vi "DriveStraightPECommand.vi"(9 "Fwd Bwd":dbl, 10 "Delay ms":u32=500, 11 "distance":dbl) -> ()   [LabVIEW 2014]
uses:
  Robot Global Data.vi
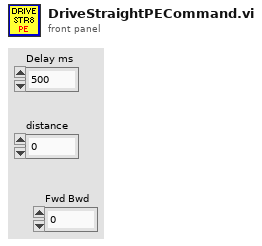
[diagram p1: front panel]
types:
  T1 = typedef "WPI_EncoderDevRef.ctl" = cluster{"DevStatus":errorcluster, "EncoderIndex":T2, "CounterIndex":T3, "DistancePerCount":dbl, "Decoding Type":T4}
  T2 = typedef "FPGA_EncoderIdx.ctl" = enum8{"Enc 0", "Enc 1", "Enc 2", "Enc 3", "Enc 4", "Enc 5", "Enc 6", "Enc 7", "Invalid"}
  T3 = typedef "FPGA_CounterCtrSystemIndex.ctl" = enum8{"Ctr 0", "Ctr 1", "Ctr 2", "Ctr 3", "Ctr 4", "Ctr 5", "Ctr 6", "Ctr 7", "Invalid"}
  T4 = typedef "WPI_EncoderType.ctl" = enum16{"1x", "2x", "4x"}
  T5 = typedef "WPI_GyroDevRef.ctl" = cluster{"DevStatus":errorcluster, "Analog Module":T6, "Analog Channel":T7, "Offset":dbl, "Gain (VoltsPerDegree/Second)":dbl}
  T6 = typedef "FPGA_TypedefAnalogModule.ctl" = enum16{"Controller 1"}
  T7 = typedef "FPGA_AIChannel.ctl" = enum8{"AI 0", "AI 1", "AI 2", "AI 3", "AI MXP 0", "AI MXP 1", "AI MXP 2", "AI MXP 3", "Invalid"}
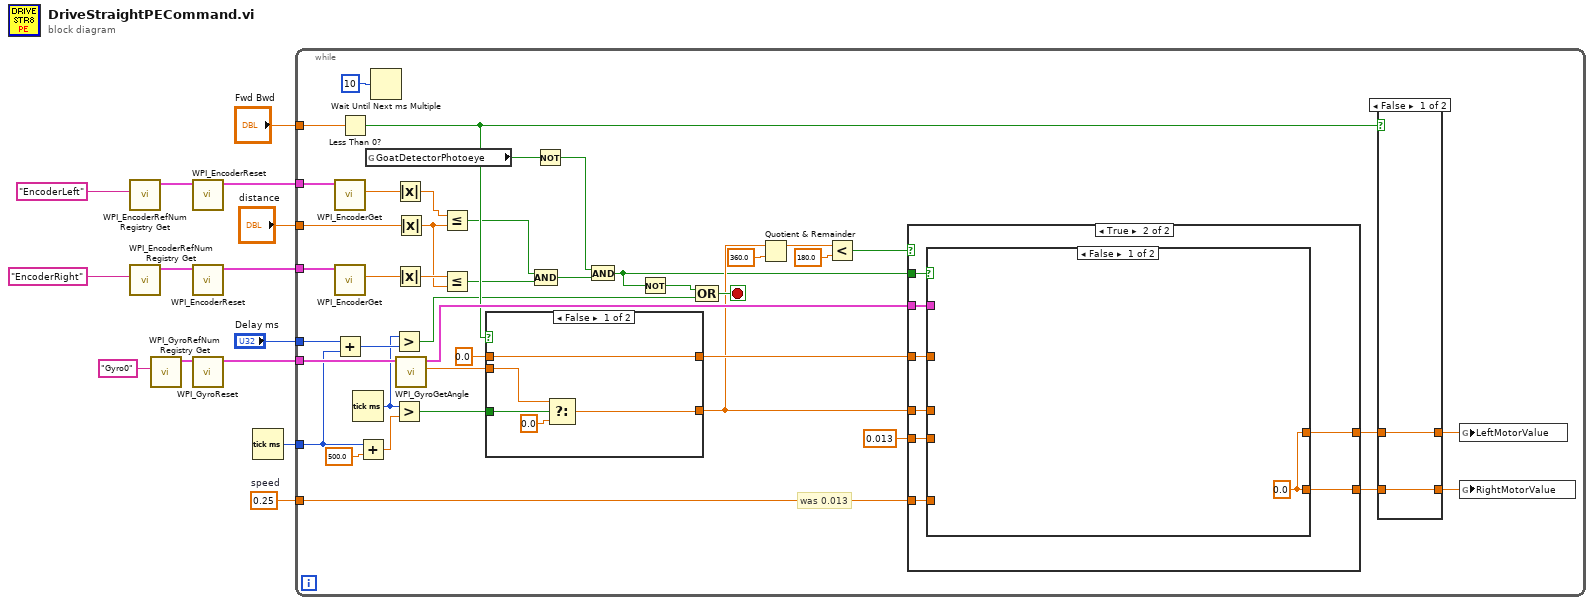
[diagram p0: block diagram]
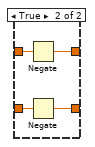
[diagram p2: hidden frame]
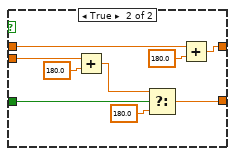
[diagram p3: hidden frame]
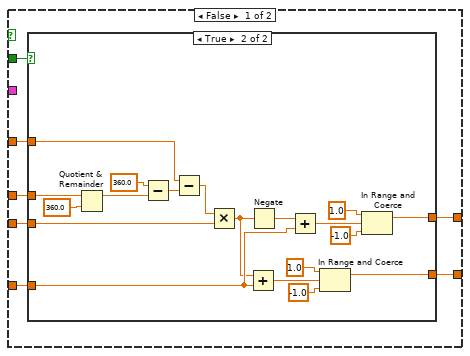
[diagram p4: hidden frame]
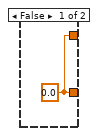
[diagram p5: hidden frame]
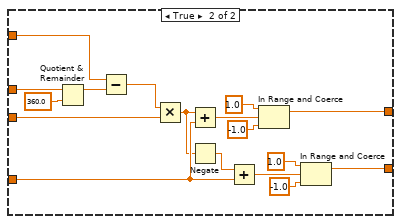
[diagram p6: hidden frame]
diagram:
  w3 = 0.25  # speed
  n1 = call <vilib>:"WPI_EncoderRefNum Registry Get.vi"("refnum name"="EncoderLeft") -> ("EncoderDevRef"=w13:T1)  [unwired: 9 in, 1 out]
  n2 = call <vilib>:"WPI_EncoderRefNum Registry Get.vi"("refnum name"="EncoderRight") -> ("EncoderDevRef"=w12:T1)  [unwired: 9 in, 1 out]
  n3 = call <vilib>:"WPI_GyroRefNum Registry Get.vi"("refnum name"="Gyro0") -> ("GyroDevRef"=w5:T5)  [unwired: 9 in, 1 out]
  n4 = call <vilib>:"WPI_EncoderReset.vi"("EncoderDevRef"=w13) -> ("EncoderDevRef"=w8:T1)  [unwired: 9 in, 1 out]
  n5 = call <vilib>:"WPI_EncoderReset.vi"("EncoderDevRef"=w12) -> ("EncoderDevRef"=w7:T1)  [unwired: 9 in, 1 out]
  n6 = call <vilib>:"WPI_GyroReset.vi"("GyroDevRef"=w5) -> ("GyroDevRef"=w4:T5)  [unwired: 9 in, 1 out]
  n7 = Tick Count (ms)() -> (millisecond timer value=w1:u32)
  n8 = while {
    tunnel: w3 -> [w50]
    tunnel: "distance" -> [w38]
    tunnel: w4 -> [w44]
    tunnel: w8 -> [w43]
    tunnel: w7 -> [w42]
    tunnel: "Fwd Bwd" -> [w41]
    tunnel: "Delay ms" -> [w27]
    tunnel: w1 -> [w25]
    stop <- w39 stop-if-true
    # "was 0.013"
    n9 = call <vilib>:"WPI_EncoderGet.vi"("EncoderDevRef"=w43) -> ("Distance"=w51:dbl)  [unwired: 5 in, 5 out]
    n10 = call <vilib>:"WPI_EncoderGet.vi"("EncoderDevRef"=w42) -> ("Distance"=w55:dbl)  [unwired: 5 in, 5 out]
    n11 = Add(x=w27, y=w25) -> (x+y=w29:u32)
    n12 = Less Than 0?(x=w41) -> (x < 0?=w35:bool)
    n13 = Tick Count (ms)() -> (millisecond timer value=w23:u32)
    n14 = Add(x=w25, y=500.0) -> (x+y=w24:dbl)
    n15 = global read "Robot Global Data.vi" "GoatDetectorPhotoeye"() -> (w21:bool)
    n16 = Wait Until Next ms Multiple(millisecond multiple=u32 10 ("milliseconds to wait")) -> ()  [unwired: 1 out]
    n17 = Greater?(x=w23, y=w29) -> (0:w28:bool)
    n18 = Greater?(x=w23, y=w24) -> (0:w22:bool)
    n19 = Absolute Value(x=w51) -> (abs(x)=w15:dbl)
    n20 = Absolute Value(x=w55) -> (abs(x)=w57:dbl)
    n21 = Absolute Value(x=w38) -> (abs(x)=w56:dbl)
    n22 = call <vilib>:"WPI_GyroGetAngle.vi"("GyroDevRef"=w44) -> ("Angle"=w52:dbl, "GyroDevRef"=w48:T5)  [unwired: 7 in, 2 out]
    n23 = Less Or Equal?(x=w15, y=w56) -> (x <= y?=w17:bool)
    n24 = Less Or Equal?(x=w57, y=w56) -> (x <= y?=w16:bool)
    n25 = case shown="False" w35 {
      tunnel: w52 -> [w67 w77]
      tunnel: [w66 w71] -> w37
      tunnel: 0.0 ("wanted angle") -> [w68 w73]
      tunnel: [w68 w75] -> w54
      tunnel: w22 -> [w65 w70]
      frame False {
        n26 = Select(t=w67, s=w65, f=0.0) -> (s? t:f=w66:dbl)
      }
      frame True {
        n27 = Add(x=w77, y=180.0) -> (x+y=w72:dbl)
        n28 = Select(t=w72, s=w70, f=180.0) -> (s? t:f=w71:dbl)
        n29 = Add(x=w73, y=180.0) -> (x+y=w75:dbl)
      }
    }
    n30 = Not(x=w21) -> (.not. x?=w19:bool)
    n31 = Compound Arithmetic op=AND(w17, w16) -> (w20:bool)
    n32 = And(x=w19, y=w20) -> (x .and. y?=w18:bool)
    n33 = Not(x=w18) -> (.not. x?=w40:bool)
    n34 = Compound Arithmetic op=OR(w40, w28) -> (w39:bool)
    n35 = Quotient & Remainder(x=w37, y=360.0) -> (x-y*floor(x/y)=w45:dbl)  [unwired: 1 out]
    n36 = Less?(x=w45, y=180.0) -> (x < y?=w34:bool)
    n37 = case shown="True" w34 {
      tunnel: w54 -> [w83 w112]
      tunnel: [w79 w106] -> w31
      tunnel: w50 -> [w84 w111]
      tunnel: 0.013 ("Kp Gain") -> [w81 w110]
      tunnel: w18 -> [w80 w109]
      tunnel: [w78 w105] -> w30
      tunnel: w48 -> [_ w108]
      tunnel: w37 -> [w82 w107]
      frame False {
        n38 = case shown="True" w80 {
          tunnel: w84 -> [_ w92]
          tunnel: w83 -> [_ w97]
          tunnel: w82 -> [_ w96]
          tunnel: w81 -> [_ w91]
          tunnel: [w85 w87] -> w78
          tunnel: [w85 w86] -> w79
          frame False {
            w85 = 0.0
          }
          frame True {
            n39 = Quotient & Remainder(x=w96, y=360.0) -> (x-y*floor(x/y)=w94:dbl)  [unwired: 1 out]
            n40 = Subtract(x=360.0, y=w94) -> (x-y=w93:dbl)
            n41 = Subtract(x=w97, y=w93) -> (x-y=w88:dbl)
            n42 = Multiply(x=w88, y=w91) -> (x*y=w89:dbl)
            n43 = Add(x=w89, y=w92) -> (x+y=w101:dbl)
            n44 = Negate(x=w89) -> (-x=w90:dbl)
            n45 = Add(x=w90, y=w92) -> (x+y=w98:dbl)
            n46 = In Range and Coerce(upper limit=1.0, x=w101, lower limit=-1.0) -> (coerced(x)=w87:dbl)  [unwired: 1 out]
            n47 = In Range and Coerce(upper limit=1.0, x=w98, lower limit=-1.0) -> (coerced(x)=w86:dbl)  [unwired: 1 out]
          }
        }
      }
      frame True {
        n48 = case shown="False" w109 {
          tunnel: w108 -> [_ _]
          tunnel: w112 -> [_ w127]
          tunnel: [w113 w115] -> w106
          tunnel: w111 -> [_ w120]
          tunnel: w110 -> [_ w124]
          tunnel: [w113 w114] -> w105
          tunnel: w107 -> [_ w121]
          frame False {
            w113 = 0.0 ("output")
          }
          frame True {
            n49 = Quotient & Remainder(x=w121, y=360.0) -> (x-y*floor(x/y)=w128:dbl)  [unwired: 1 out]
            n50 = Subtract(x=w127, y=w128) -> (x-y=w116:dbl)
            n51 = Multiply(x=w116, y=w124) -> (x*y=w119:dbl)
            n52 = Add(x=w119, y=w120) -> (x+y=w125:dbl)
            n53 = Negate(x=w119) -> (-x=w117:dbl)
            n54 = Add(x=w117, y=w120) -> (x+y=w118:dbl)
            n55 = In Range and Coerce(upper limit=1.0, x=w125, lower limit=-1.0) -> (coerced(x)=w115:dbl)  [unwired: 1 out]
            n56 = In Range and Coerce(upper limit=1.0, x=w118, lower limit=-1.0) -> (coerced(x)=w114:dbl)  [unwired: 1 out]
          }
        }
      }
    }
    n57 = case shown="False" w35 {
      tunnel: [w59 w62] -> w33
      tunnel: [w58 w63] -> w32
      tunnel: w31 -> [w59 w61]
      tunnel: w30 -> [w58 w60]
      frame False {
      }
      frame True {
        n58 = Negate(x=w61) -> (-x=w62:dbl)
        n59 = Negate(x=w60) -> (-x=w63:dbl)
      }
    }
    n60 = global write "Robot Global Data.vi" "LeftMotorValue"(w33) -> ()
    n61 = global write "Robot Global Data.vi" "RightMotorValue"(w32) -> ()
  }
